vi "RPC Get Component Version.vi"(8 "error in (no error)":errorcluster, 9 "Component (\"\")":string, 10 "Component Library (empty)":path, 11 "app reference (empty)":refnum<vi>) -> (0 "error out":errorcluster, 1 "Component Version":cluster{"Version":string, "Build Number":u32}, 2 "vi ref valid?":bool, 3 "app reference":refnum<vi>)   [LabVIEW 2011]
uses:
  Summitek EXT/Miscellaneous/OGAB Version.ctl
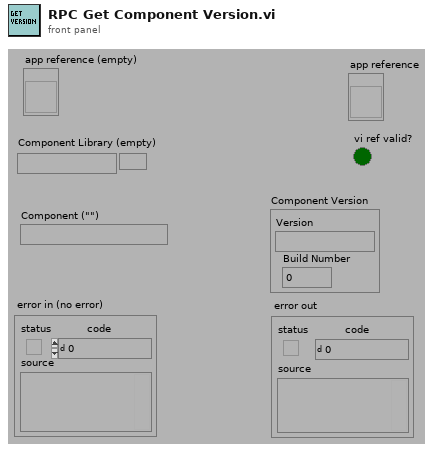
[diagram p1: front panel]
types:
  T1 = enum32{"invalid app kind", "Development System", "Run Time System", "Student Edition", "Embedded LabVIEW", "Evaluation", "Custom"}
  T2 = typedef "OGAB Version.ctl" = cluster{"Version":string, "Build Number":u32, "Build Date/Time":dbl}
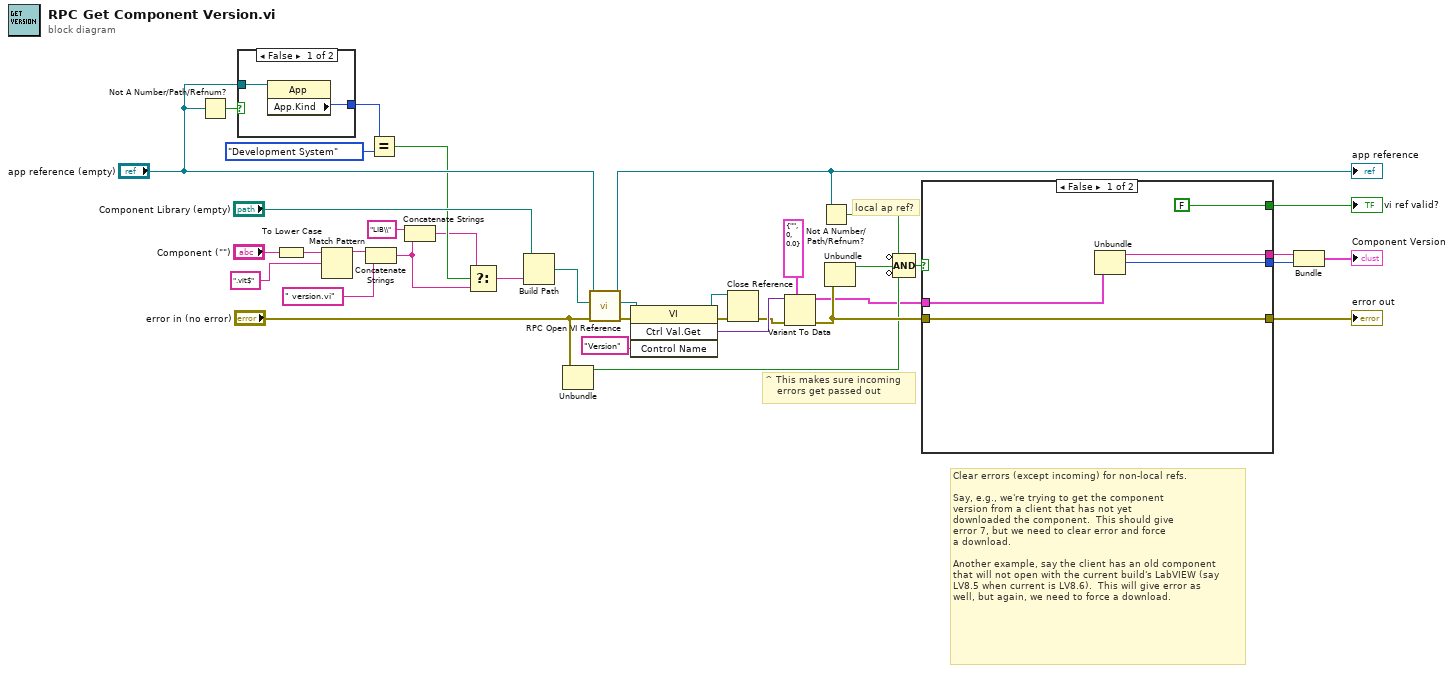
[diagram p0: block diagram]
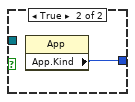
[diagram p2: hidden frame]
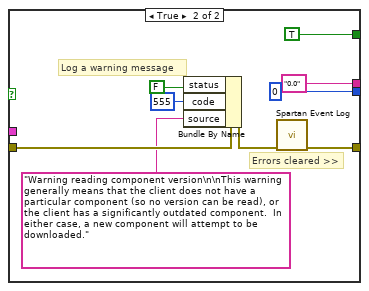
[diagram p3: hidden frame]
diagram:
  # "^ This makes sure incoming\n    errors get passed out"
  # "local ap ref?"
  # "Clear errors (except incoming) for non-local refs.\n\nSay, e.g., we're trying to get the component\nversion from a client that has not yet\ndownloaded the component.  This should give\nerror 7, but we need to clear error and force\na download.\n\nAnother example, say the client has an old component \nthat will not open with the current build's LabVIEW (say\nLV8.5 when current is LV8.6).  This will give error as\nwell, but again, we need to force a download."
  n1 = Not A Number/Path/Refnum?(number/path/refnum="app reference (empty)") -> (NaN/Path/Refnum?=w6:bool)
  n2 = case shown="False" w6 {
    tunnel: [w39 w40] -> w21
    tunnel: "app reference (empty)" -> [w38 _]
    frame False {
      n3 = property class="App"(reference=w38) -> ("App.Kind"=w39:T1)  [unwired: 1 in, 2 out]
    }
    frame True {
      n4 = property class="App"() -> ("App.Kind"=w40:T1)  [unwired: 2 in, 2 out]
    }
  }
  n5 = To Lower Case(string="Component (\"\")") -> (all lower case string=w27:string)
  n6 = Match Pattern(string=w27, regular expression=".vit$" ("search string")) -> (before substring=w24:string)  [unwired: 1 in, 3 out]
  n7 = Concatenate Strings(w24, " version.vi" ("replace string (\"\")")) -> (w16:string)
  n8 = Equal?(x=w21, y=T1."Development System") -> (x = y?=w19:bool)
  n9 = Concatenate Strings("LIB\\" ("string"), w16) -> (w18:string)
  n10 = Select(t=w18, s=w19, f=w16) -> (s? t:f=w17:string)
  n11 = Build Path(base path="Component Library (empty)", name or relative path=w17) -> (appended path=w28:path)
  n12 = Unbundle("error in (no error)") -> ("status"=w5:bool)  [unwired: 2 out]
  n13 = call "RPC Open VI Reference.vi"("error in (no error)"="error in (no error)", "VI path (empty)"=w28, "app reference (empty)"="app reference (empty)") -> ("error out"=w1:errorcluster, "vi reference"=w14:refnum<vi>, "dup app reference"=w34:refnum<vi>)  [unwired: 6 out]
  "app reference" <- w34
  n14 = invoke class="VI" method="Ctrl Val.Get"(reference=w14, error in=w1, "Control Name"="Version") -> (reference out=w25:refnum<vi>, error out=w10:errorcluster, "Get Control Value Variant"=w15:variant)  [unwired: 1 in, 1 out]
  n15 = Close Reference(reference=w25, error in (no error)=w10) -> (error out=w9:errorcluster)
  n16 = Variant To Data(error in=w9, type=T2 {"Version"="", "Build Number"=0, "Build Date/Time"=0.0} ("Version"), Variant=w15) -> (data=w4:T2, error out=w8:errorcluster)
  n17 = Not A Number/Path/Refnum?(number/path/refnum=w34) -> (NaN/Path/Refnum?=w11:bool)
  n18 = Unbundle(w8) -> ("status"=w12:bool)  [unwired: 2 out]
  n19 = Compound Arithmetic op=AND(invert w11, w12, invert w5) -> (w7:bool)
  n20 = case shown="False" w7 {
    tunnel: w8 -> [w45 w48]
    tunnel: [w45 w47] -> w33
    tunnel: w4 -> [w44 _]
    tunnel: [w43 "0.0" ("Version")] -> w3
    tunnel: [w42 u32 0 ("Build Number")] -> w2
    tunnel: [FALSE TRUE] -> w31
    frame False {
      n21 = Unbundle(w44) -> ("Version"=w43:string, "Build Number"=w42:u32)  [unwired: 1 out]
    }
    frame True {
      # "Errors cleared >>"
      # "Log a warning message"
      n22 = Bundle By Name(cluster=w48, "status"=FALSE, "code"=555, "source"="Warning reading component version\n\nThis warning generally means that the client does not have a particular component (so no version can be read), or the client has a significantly outdated component.  In either case, a new component will attempt to be downloaded." ("name (unnamed)")) -> (w51:errorcluster)
      n23 = call "Spartan Event Log.vi"("error in (no error)"=w51) -> ("error out"=w47:errorcluster)  [unwired: 7 in]
    }
  }
  "error out" <- w33
  "vi ref valid?" <- w31
  n24 = Bundle("Version"=w3, "Build Number"=w2) -> (→"Component Version":cluster{"Version":string, "Build Number":u32})  [unwired: 1 out]
